vi "Create New File.vi"(8 "error in":errorcluster) -> (0 "error out":errorcluster, 3 "File Directory":T1)   [LabVIEW 2025, in "Control de MaP.lvlib"]
uses:
  Control de MaP.lvlib
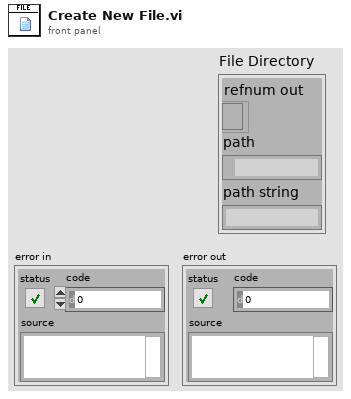
[diagram p1: front panel]
types:
  T1 = cluster{"refnum out":refnum<file>, "path":path, "path string":string}
  T2 = enum16{"open", "replace", "create", "open or create", "replace or create", "replace or create with confirmation"}
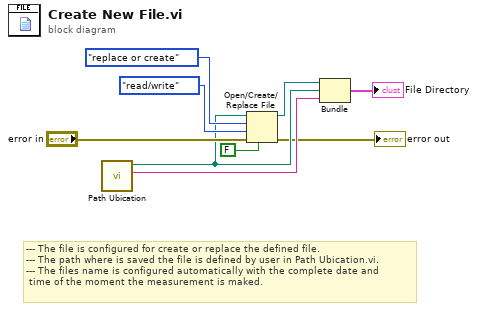
[diagram p0: block diagram]
diagram:
  # "--- The file is configured for create or replace the defined file.\n--- The path where is saved the file is defined by user in Path Ubication.vi.\n--- The files name is configured automatically with the complete date and\n time of the moment the measurement is maked."
  n1 = call "Path Ubication.vi"() -> ("path string"=w4:string, "path"=w5:path)  [unwired: 8 in]
  n2 = Open/Create/Replace File(file path (use dialog)=w5, error in="error in", operation (0:open)=T2."replace or create", access (0:read/write)=enum16{"read/write", "read-only", "write-only"}."read/write", disable buffering (F)=FALSE) -> (refnum out=w1:refnum<file>, error out=→"error out":errorcluster)  [unwired: 1 in, 1 out]
  n3 = Bundle("refnum out"=w1, "path"=w5, "path string"=w4) -> (→"File Directory":T1)  [unwired: 1 in]
